vi "DC Voltage Source.vi"() -> ()   [LabVIEW 2017]
panel:
  out "error out":errorcluster
  in  "Numeric":dbl format="%.4g"
  in  "stop":bool
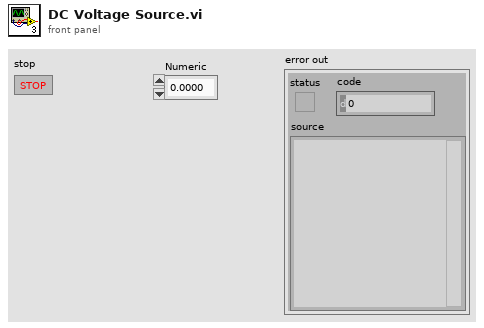
[diagram p1: front panel]
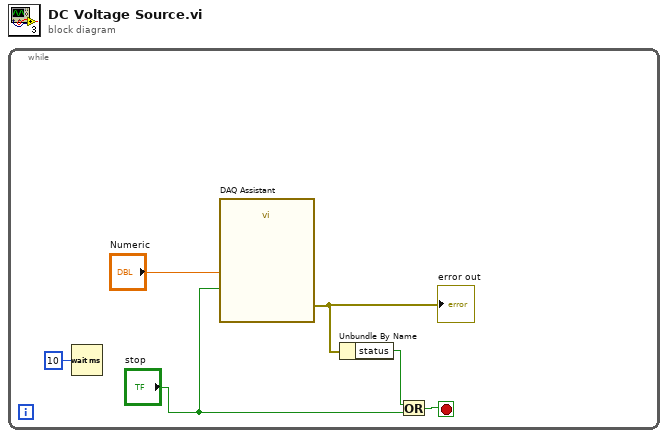
[diagram p0: block diagram]
diagram:
  n1 = while {
    stop <- w1 stop-if-true
    n2 = Wait (ms)(milliseconds to wait=u32 10) -> ()  [unwired: 1 out]
    n3 = call "DAQ Assistant"("data"="Numeric", "stop (T)"="stop") -> ("error out"=w4:errorcluster)  [unwired: 16 in, 1 out]
    "error out" <- w4
    n4 = Unbundle By Name "Unbundle By Name"(w4) -> ("status"=w2:bool)
    n5 = Or(x=w2, y="stop") -> (x .or. y?=w1:bool)
  }
